vi "CSM - Running Log(Auto Filter Loop State) - DebugTool.vi"() -> ()   [LabVIEW 2017]
uses:
  _Support/Typedef/_CSM_GlobalLog_MSG.ctl
  _Support/Typedef/_CSM_Response Source Message.ctl
  _Support/Typedef/_CSM_GlobalLog_MSG_TYPE.ctl
  _Support/GlobalEvent/Gevt-ThreadQueueName.vi
  _Support/FGV-BroadcastRegistry/global-CSMQ FGV Change Flag.vi
  _Support/CSMQ/_CSMOFGV.vi
  Communicable State Machine.lvlib
  _Support/csm-tool-support.lvlib
  addons/Logger/CSM File Logger.lvlib
panel:
  in  "Record.Stop":bool
  in  "Record.Start":bool
  in  "BackTop":bool
  in  "Toolbar.History Length(char)":i32=100000 caption="History(char)" min=1000 max=100000000 step=1
  in  "Clear":bool
  in  "CSM":string(combo)
  in  "Search Button":bool
  in  "Toolbar.Open BD":bool
  in  "Toolbar.Open FP":bool
  out "State History":string
  in  "Tab":enum32{"Error History", "Broadcast Registry"}(tab)
  out "Error History":string
  out "Broadcast Registry":string[][](table)
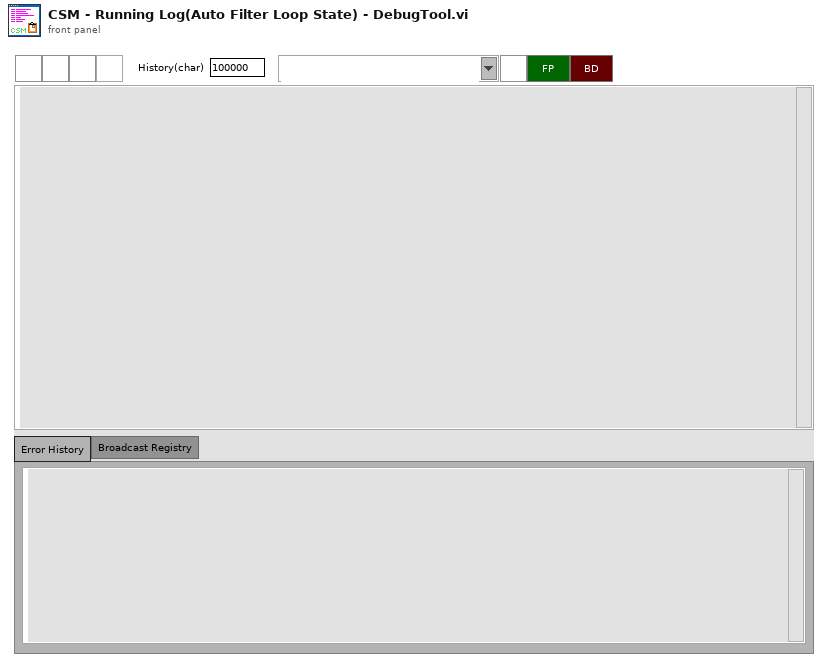
[diagram p1: front panel]
types:
  T1 = typedef "Communicable State Machine.lvlib/_CSM_GlobalLog_MSG.ctl" = cluster{"Name(\"\" to use uuid)":string, "Current State":string, "Arguments":string, "Source Message":T2, "Source Module":string, "Complete(T)/Start(F)":bool, "LogType":T3}
  T2 = typedef "Communicable State Machine.lvlib/_CSM_Response Source Message.ctl" = cluster{"‘State":string, "’Arguments":string, "’Error":errorcluster}
  T3 = typedef "Communicable State Machine.lvlib/_CSM_GlobalLog_MSG_TYPE.ctl" = enum16{"User Log", "State Change", "Status", "Interrupt", "Register", "Unregister", "Error Log", "Module Created", "Module Destroyed"}
  T4 = enum32{"Invalid", "Standard", "Closed", "Hidden", "Minimized", "Maximized"}
  T5 = enum32{"invalid app kind", "Development System", "Run Time System", "Student Edition", "Embedded LabVIEW", "Evaluation", "Custom"}
  T6 = cluster{"Shift":bool, "Ctrl":bool, "Alt":bool, "Cmd":bool, "Opt":bool}
  T7 = cluster{"Core":cluster{"Current VI Reference":refnum<vi>, "Close Panel on Exit?":bool}, "Toolbar.Advance":refnum<vi>[], "LoggerWatchDogQueue":refnum<queue>, "LogFile":path}
  T8 = cluster{"Current VI Reference":refnum<vi>, "Close Panel on Exit?":bool}
  T9 = typedef "Communicable State Machine.lvlib/CSM - Broadcast Message Type.ctl" = enum16{"Status", "Interrupt(High)"}
  T10 = cluster{"Status":string, "Source CSM":string, "Target CSM":string, "Target API":string, "Priority":T9}[]
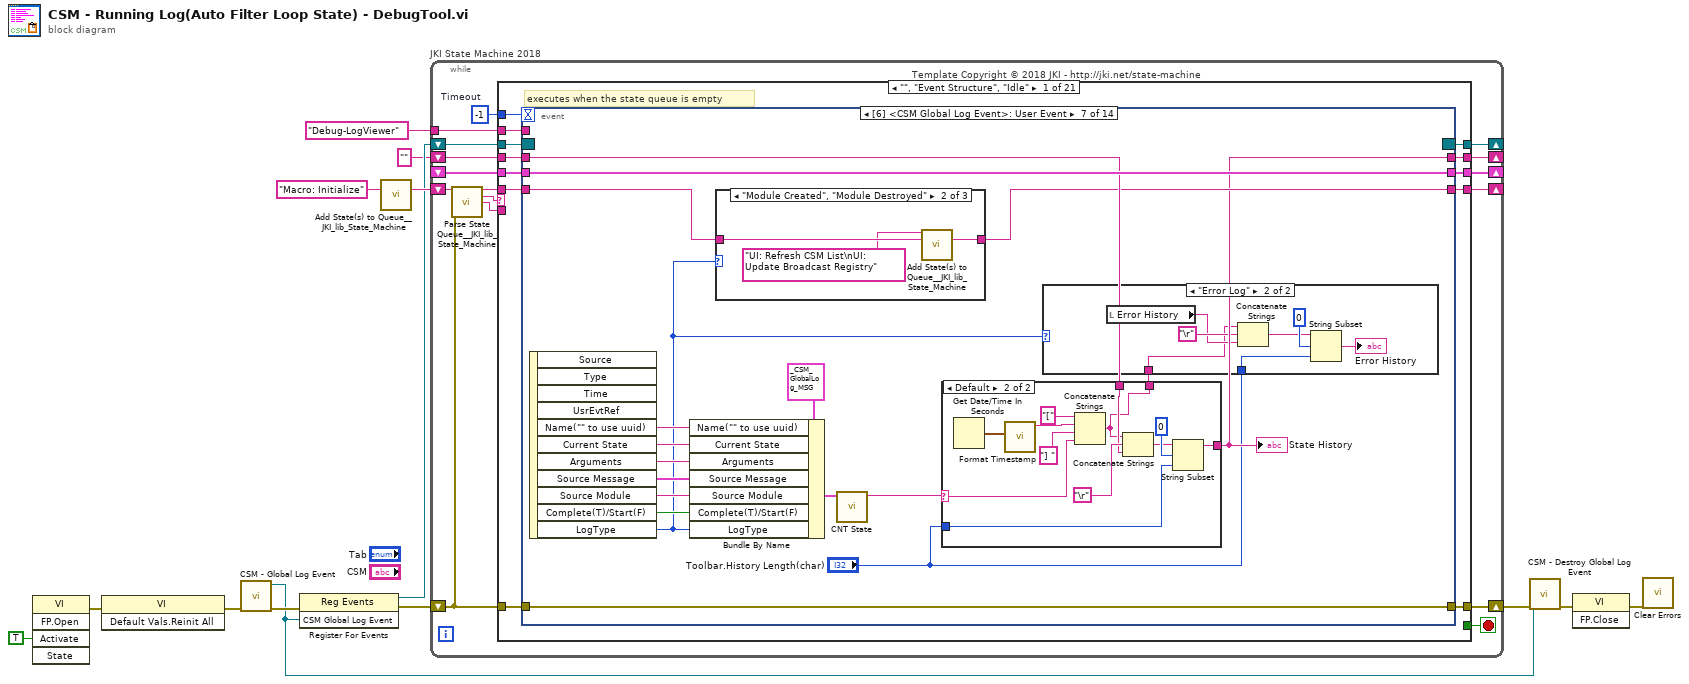
[diagram p0: block diagram]
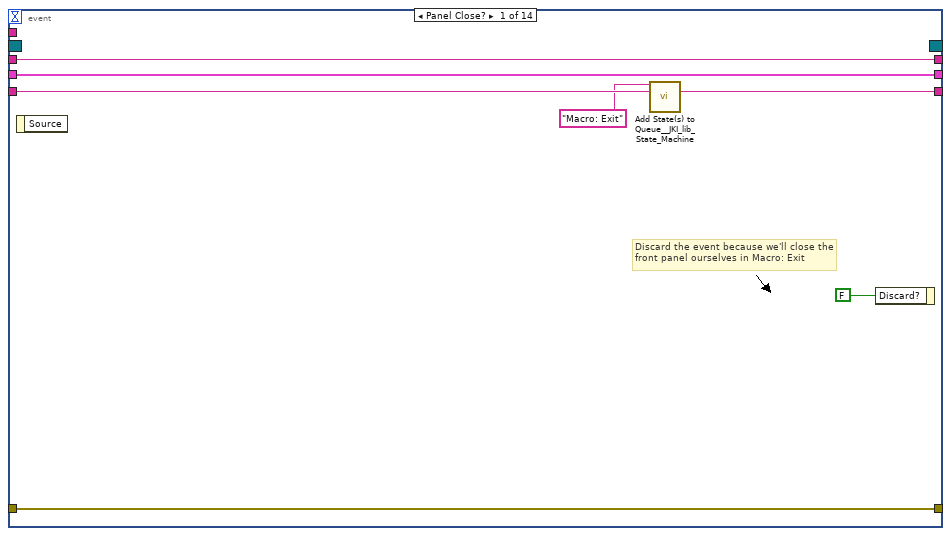
[diagram p2: hidden frame]
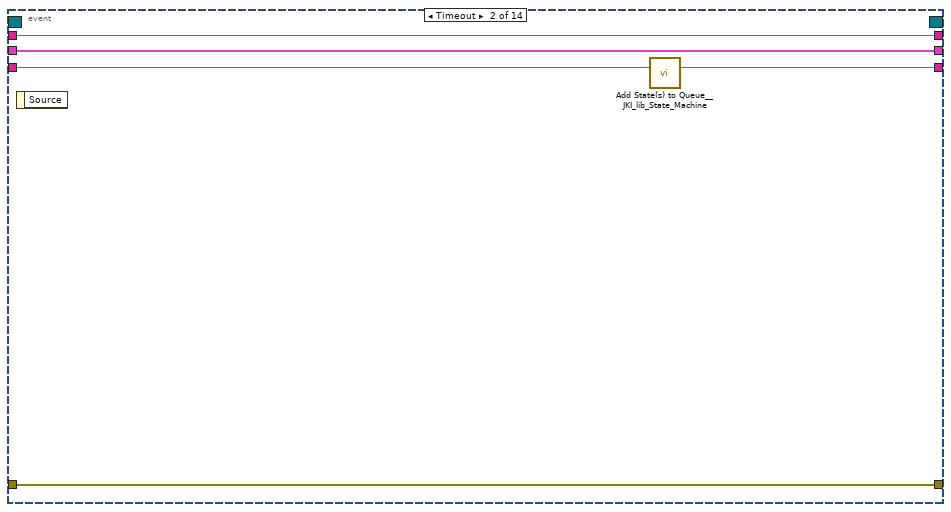
[diagram p3: hidden frame]
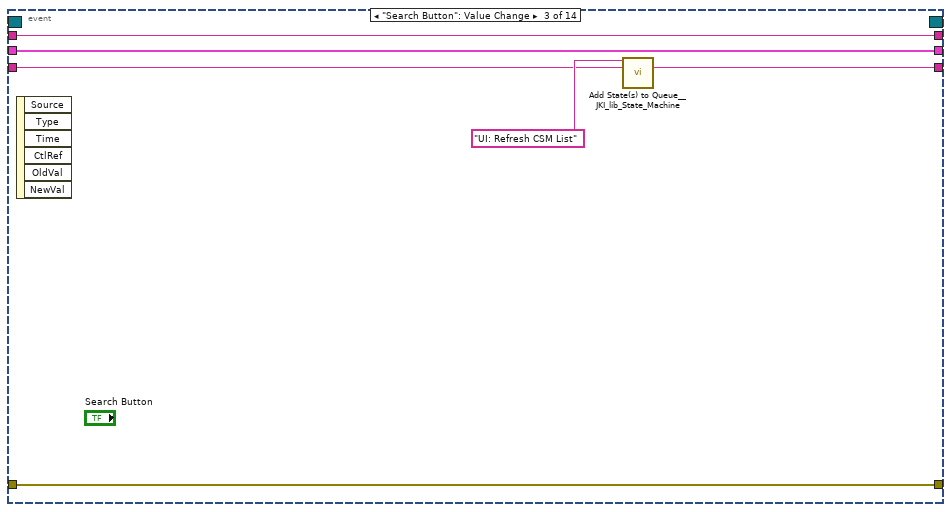
[diagram p4: hidden frame]
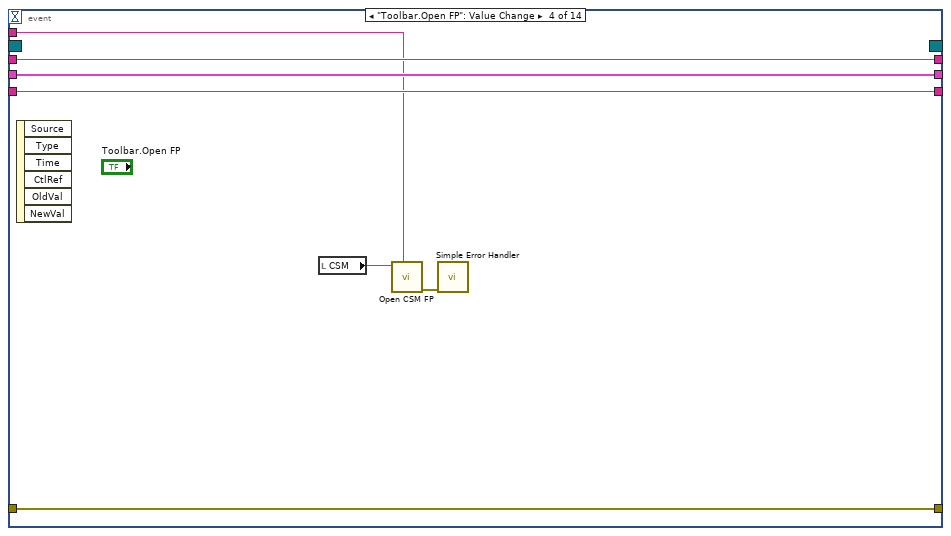
[diagram p5: hidden frame]
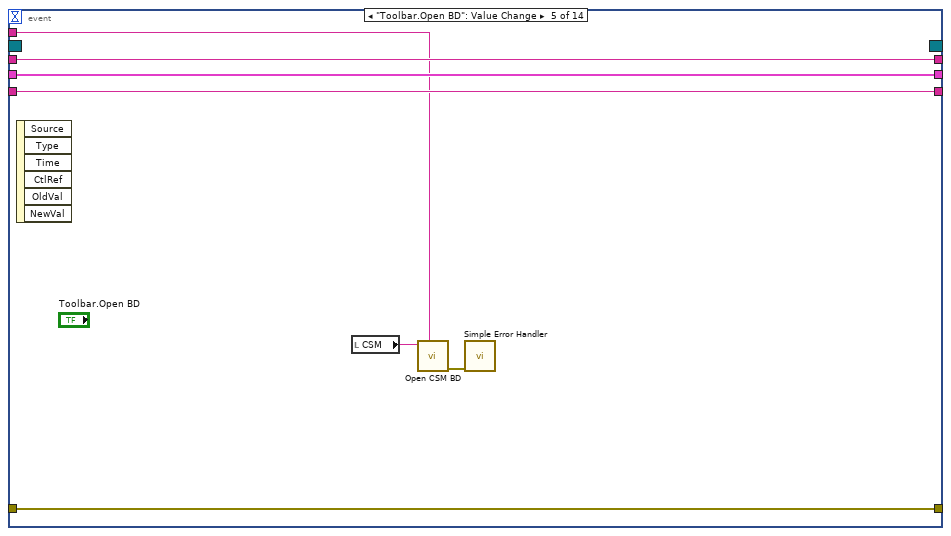
[diagram p6: hidden frame]
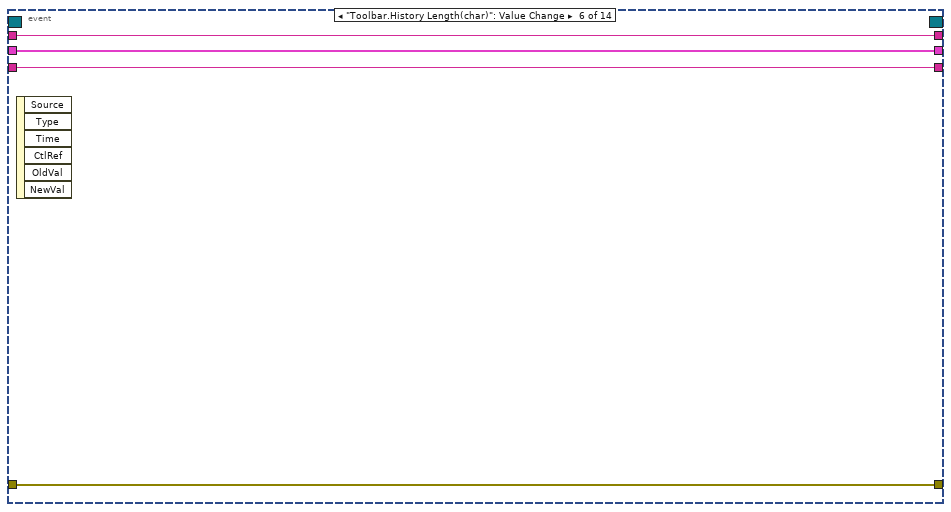
[diagram p7: hidden frame]
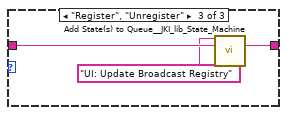
[diagram p10: hidden frame]
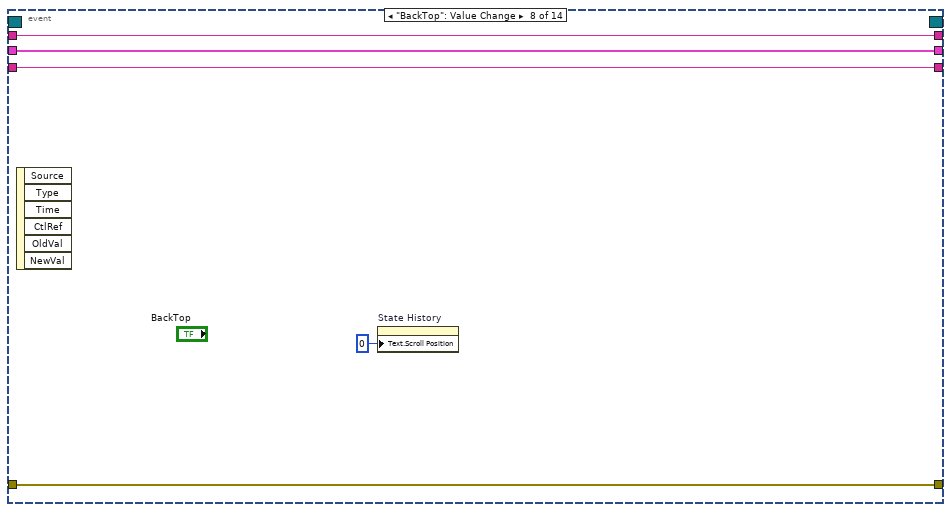
[diagram p12: hidden frame]
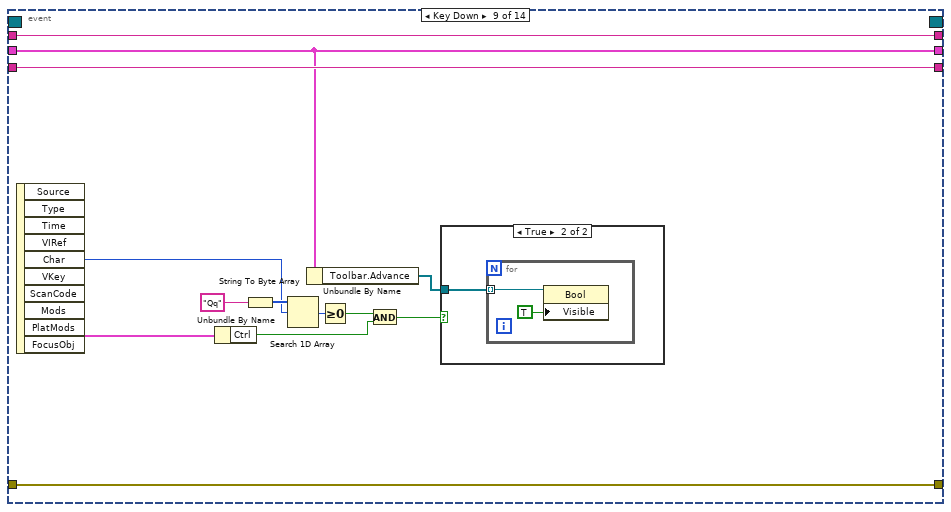
[diagram p13: hidden frame]
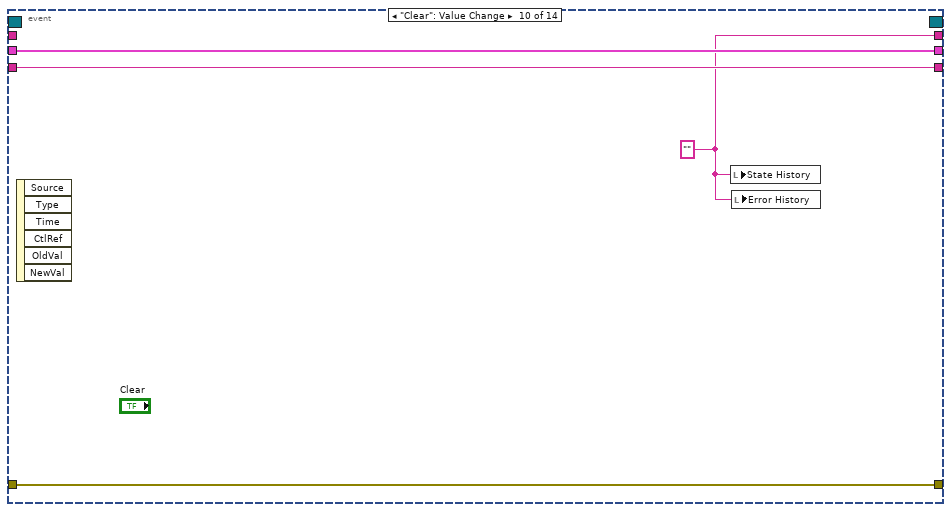
[diagram p15: hidden frame]
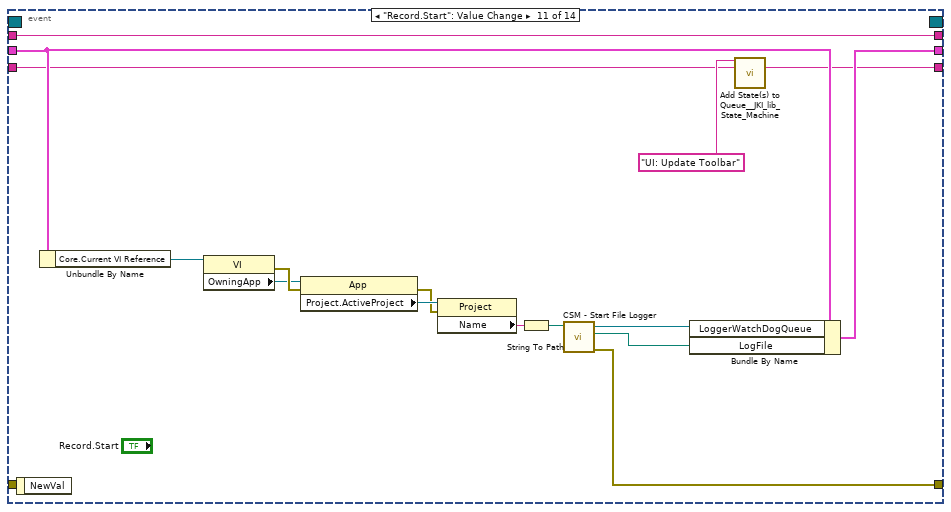
[diagram p16: hidden frame]
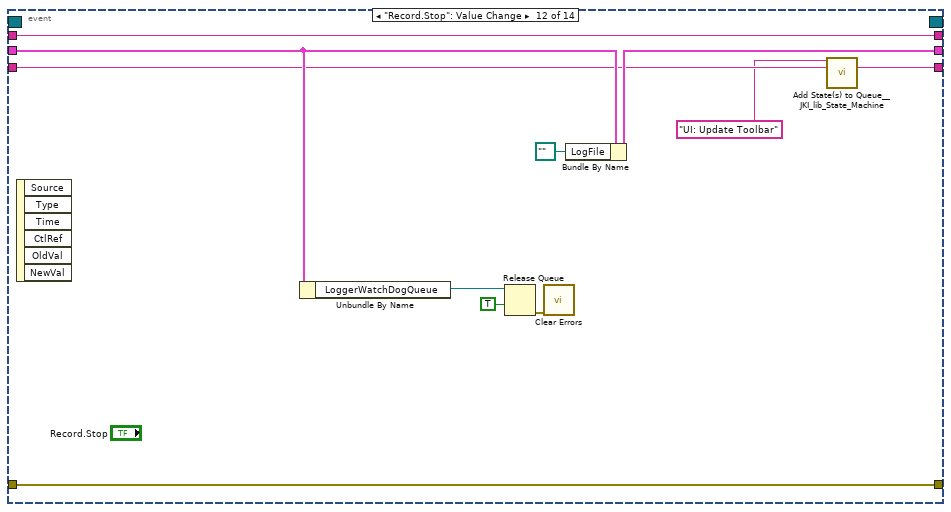
[diagram p17: hidden frame]
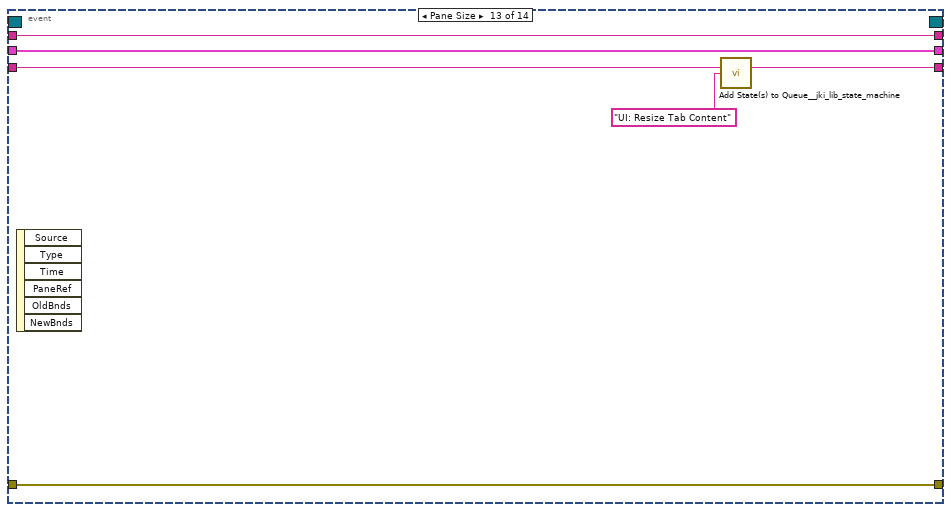
[diagram p18: hidden frame]
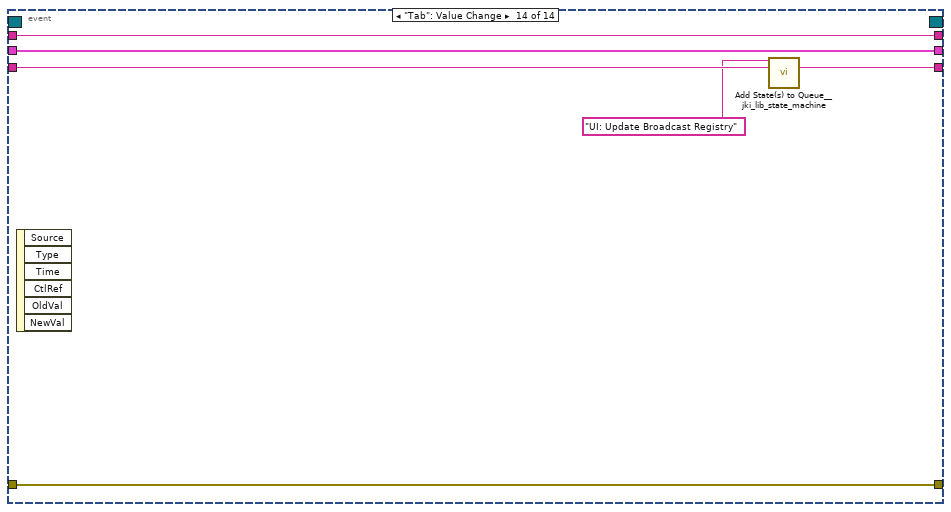
[diagram p19: hidden frame]
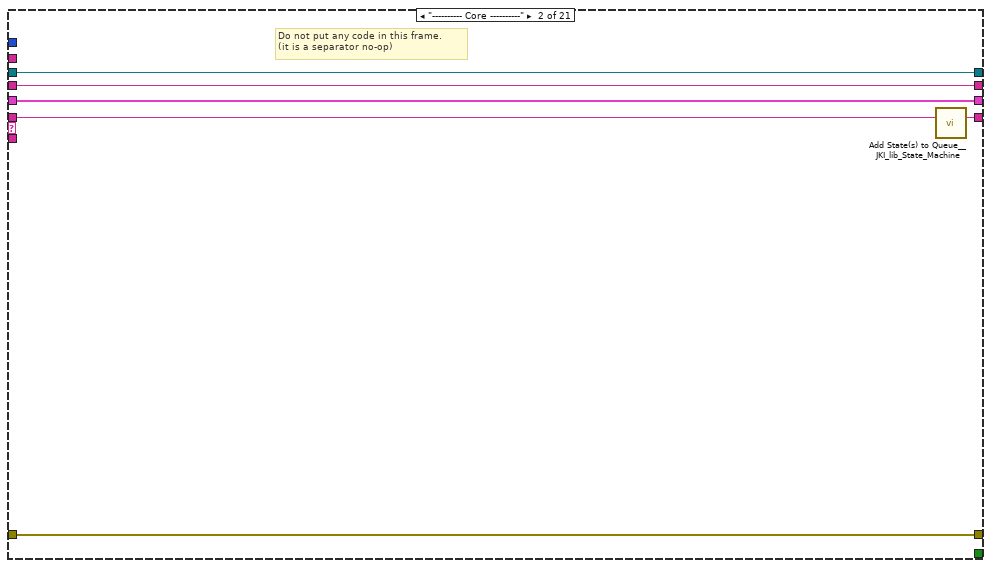
[diagram p20: hidden frame]
diagram:
  n1 = invoke class="VI" method="FP.Open"("Activate"=TRUE ("Activate?")) -> (error out=w13:errorcluster)  [unwired: 4 in, 4 out]
  n2 = invoke class="VI" method="Default Vals.Reinit All"(error in=w13) -> (error out=w7:errorcluster)  [unwired: 2 in, 2 out]
  n3 = call "CSM - Global Log Event.vi"("Error in"=w7) -> ("Error out"=w11:errorcluster, "CSM Global Log Event"=w10:refnum<user-event>)  [unwired: 9 in]
  n4 = register-events(error in=w11, w10) -> (reference out=w5:refnum<event-registration>, error out=w6:errorcluster)  [unwired: 1 in]
  n5 = call <vilib>:"Add State(s) to Queue__JKI_lib_State_Machine.vi"("State(s) in (\"\")"="Macro: Initialize") -> ("States Out"=w9:string)  [unwired: 14 in]
  n6 = while "JKI State Machine 2018" {
    shift-right: [w23] -> _
    shift-left: _ -> [w22]
    shift-right: [w26] -> w4
    shift-left: w6 -> [w20]
    shift-right: [w25] -> _
    shift-left: w9 -> [w27]
    shift-right: [w18] -> _
    shift-left: w5 -> [w19]
    tunnel: "Debug-LogViewer" ("Current Module(\"\" to generate a ID)") -> [w17]
    shift-right: [w15] -> _
    shift-left: "" ("String Cache") -> [w16]
    stop <- w24 stop-if-true
    w21 = -1  # Timeout
    # "Template Copyright © 2018 JKI - http://jki.net/state-machine"
    n7 = call <vilib>:"Parse State Queue__JKI_lib_State_Machine.vi"("State Queue"=w27, "Error In (no error)"=w20) -> ("Remaining States"=w29:string, "Current State"=w30:string, "Arguments"=w28:string)  [unwired: 11 in]
    n8 = case shown="\"\", \"Event Structure\", \"Idle\"" w30 {
      selector: w30 -> [_ _ w196 _ _ _ _ _ _ _ _ _ _ _ _ _ _ _ _ _ _]
      tunnel: w29 -> [w42 w193 w200 w221 w229 w236 w242 w252 w261 w269 w275 w282 w293 w306 w382 w389 w417 w440 w447 w454 w466]
      tunnel: w28 -> [_ _ _ _ _ _ _ _ _ _ _ _ w288 w300 _ _ _ _ _ _ _]
      tunnel: w22 -> [w40 w190 w198 w214 w226 w234 w239 _ w260 w264 w272 w277 w291 w302 w381 w388 w412 w439 w444 w451 w463]
      tunnel: [w39 w191 w202 w218 errorcluster {"status"=FALSE, "code"=0, "source"=""} ("error out") w233 w240 w249 w253 w265 w273 w280 w289 w303 w383 w390 w418 w441 w445 w452 w464] -> w26
      tunnel: w20 -> [w38 w191 w201 w218 w225 w233 w240 w249 w253 w266 w273 w280 w290 w304 w383 w390 w418 w441 w445 w452 w464]
      tunnel: [w41 w192 w199 w220 w228 w235 w241 w251 w261 w268 w274 w281 w292 w305 w382 w389 w417 w440 w446 w453 w465] -> w25
      tunnel: [_ _ _ _ _ TRUE _ _ _ _ _ _ _ _ _ _ _ _ _ _ _] -> w24
      tunnel: [w37 w190 w198 w219 w226 w234 w239 w250 w257 w264 w272 w277 w291 w302 w381 w388 w412 w439 w444 w451 w463] -> w23
      tunnel: w21 -> [w36 _ _ _ _ _ _ _ _ _ _ _ _ _ _ _ _ _ _ _ _]
      tunnel: w19 -> [w35 w189 w195 w208 w223 w231 w238 w247 w259 w263 w271 w279 w287 w299 w380 w387 w416 w438 w443 w449 w456]
      tunnel: [w34 w189 w195 w208 w223 w231 w238 w247 w259 w263 w271 w279 w287 w299 w380 w387 w416 w438 w443 w449 w456] -> w18
      tunnel: w17 -> [w33 _ _ _ _ _ _ _ _ _ _ _ _ _ _ _ _ _ _ _ _]
      tunnel: w16 -> [w32 w188 w194 w207 w222 w230 w237 w246 w258 w262 w270 w278 w286 w298 w379 w386 w415 w437 w442 w448 w455]
      tunnel: [w31 w188 w194 w207 w222 w230 w237 w246 w258 w262 w270 w278 w286 w298 w379 w386 w415 w437 w442 w448 w455] -> w15
      frame "", "Event Structure", "Idle" {
        # "executes when the state queue is empty"
        n9 = event shown="[6] <CSM Global Log Event>: User Event" {
          selector: w35 -> [_ _ _ _ _ _ _ _ _ _ _ _ _ _]
          dyn-events: [_ _ _ _ _ _ _ _ _ _ _ _ _ _] -> w34
          timeout: w36 -> [_ _ _ _ _ _ _ _ _ _ _ _ _ _]
          tunnel: w42 -> [w49 w54 w56 w66 w74 w78 w86 w128 w141 w148 w150 w167 w177 w183]
          tunnel: [w48 w53 w55 w66 w74 w78 w85 w128 w141 w148 w149 w166 w178 w184] -> w41
          tunnel: w40 -> [w46 w51 w60 w67 w72 w76 w95 w126 w131 w146 w159 w173 w180 w186]
          tunnel: [w47 w52 w59 w65 w73 w77 w96 w127 w140 w147 w161 w175 w181 w187] -> w39
          tunnel: w38 -> [w47 w52 w59 w65 w73 w77 w96 w127 w140 w147 _ w175 w181 w187]
          tunnel: [w46 w51 w60 w67 w72 w76 w95 w126 w131 w146 w162 w169 w180 w186] -> w37
          tunnel: w33 -> [_ _ _ w62 w69 _ _ _ _ _ _ _ _ _]
          tunnel: w32 -> [w43 w50 w58 w64 w71 w75 w87 w125 w139 _ w164 w174 w179 w185]
          tunnel: [w43 w50 w58 w64 w71 w75 w83 w125 w139 w145 w164 w174 w179 w185] -> w31
          event Panel Close? {
            # "Discard the event because we'll close the front panel ourselves in Macro: Exit"
            n10 = event-data() -> ()  [unwired: 1 in, 1 out]
            n11 = call <vilib>:"Add State(s) to Queue__JKI_lib_State_Machine.vi"("State(s) in Front (\"\")"="Macro: Exit", "State(s) in (\"\")"=w49) -> ("States Out"=w48:string)  [unwired: 13 in]
            n12 = event-data("Discard?"=FALSE) -> ()  [unwired: 1 in, 1 out]
          }
          event Timeout {
            n13 = event-data() -> ()  [unwired: 1 in, 1 out]
            n14 = call <vilib>:"Add State(s) to Queue__JKI_lib_State_Machine.vi"("State(s) in (\"\")"=w54) -> ("States Out"=w53:string)  [unwired: 14 in]
          }
          event "Search Button": Value Change {
            n15 = event-data() -> ()  [unwired: 1 in, 6 out]
            n16 = call <vilib>:"Add State(s) to Queue__JKI_lib_State_Machine.vi"("State(s) in Front (\"\")"="UI: Refresh CSM List" ("State(s) in Front (\"\")"), "State(s) in (\"\")"=w56) -> ("States Out"=w55:string)  [unwired: 13 in]
          }
          event "Toolbar.Open FP": Value Change {
            n17 = event-data() -> ()  [unwired: 1 in, 6 out]
            n18 = local read "CSM"() -> (w61:string)
            n19 = call "Open CSM FP.vi"("Current Module(\"\" to generate a ID)"=w62, "CSM"=w61) -> ("error out"=w63:errorcluster)  [unwired: 9 in]
            n20 = call <vilib>:"Simple Error Handler.vi"("error in (no error)"=w63) -> ()  [unwired: 4 in, 5 out]
          }
          event "Toolbar.Open BD": Value Change {
            n21 = event-data() -> ()  [unwired: 1 in, 6 out]
            n22 = local read "CSM"() -> (w68:string)
            n23 = call "Open CSM BD.vi"("Current Module(\"\" to generate a ID)"=w69, "CSM"=w68) -> ("error out"=w70:errorcluster)  [unwired: 9 in]
            n24 = call <vilib>:"Simple Error Handler.vi"("error in (no error)"=w70) -> ()  [unwired: 4 in, 5 out]
          }
          event "Toolbar.History Length(char)": Value Change {
            n25 = event-data() -> ()  [unwired: 1 in, 6 out]
          }
          event User Event {
            n26 = event-data() -> ("Name(\"\" to use uuid)"=w93:string, "Current State"=w92:string, "Arguments"=w91:string, "Source Message"=w90:T2, "Source Module"=w89:string, "Complete(T)/Start(F)"=w88:bool, "LogType"=w84:T3)  [unwired: 1 in, 4 out]
            n27 = Bundle By Name(cluster=T1 {"Name(\"\" to use uuid)"="", "Current State"="", "Arguments"="", "Source Message"={"‘State"="", "’Arguments"="", "’Error"={"status"=FALSE, "code"=0, "source"=""}}, "Source Module"="", "Complete(T)/Start(F)"=FALSE, "LogType"=enum."State Change"} ("Cross CSM Data"), "Name(\"\" to use uuid)"=w93, "Current State"=w92, "Arguments"=w91, "Source Message"=w90, "Source Module"=w89, "Complete(T)/Start(F)"=w88, "LogType"=w84) -> (w80:T1)
            n28 = case shown="\"Module Created\", \"Module Destroyed\"" w84 {
              tunnel: w86 -> [w104 w107 w110]
              tunnel: [w104 w106 w109] -> w85
              frame "User Log", Default {
              }
              frame "Module Created", "Module Destroyed" {
                n29 = call <vilib>:"Add State(s) to Queue__JKI_lib_State_Machine.vi"("State(s) in Front (\"\")"="UI: Refresh CSM List\nUI: Update Broadcast Registry" ("State(s) in Front (\"\")"), "State(s) in (\"\")"=w107) -> ("States Out"=w106:string)  [unwired: 13 in]
              }
              frame "Register", "Unregister" {
                n30 = call <vilib>:"Add State(s) to Queue__JKI_lib_State_Machine.vi"("State(s) in Front (\"\")"="UI: Update Broadcast Registry" ("State(s) in Front (\"\")"), "State(s) in (\"\")"=w110) -> ("States Out"=w109:string)  [unwired: 13 in]
              }
            }
            n31 = call "CNT State.vi"("Cross CSM Data"=w80) -> ("Log String"=w79:string)  [unwired: 9 in, 1 out]
            n32 = case shown="Default" w79 {
              selector: w79 -> [_ w123]
              tunnel: [w111 w121] -> w83
              tunnel: "Toolbar.History Length(char)" -> [_ w120]
              tunnel: w87 -> [w111 w115]
              tunnel: [_ w114] -> w81
              frame "" {
              }
              frame Default {
                n33 = Get Date/Time In Seconds() -> (seconds since 1Jan1904=w112:timestamp)
                n34 = call "Format Timestamp.vi"("timestamp"=w112) -> ("String"=w113:string)  [unwired: 10 in]
                n35 = Concatenate Strings("[" ("string"), w113, "] " ("string"), w123) -> (w114:string)
                n36 = Concatenate Strings(w114, "\r", w115) -> (w117:string)
                n37 = String Subset(string=w117, offset (0)=0, length (rest)=w120) -> (substring=w121:string)
              }
            }
            "State History" <- w83
            n38 = case shown="\"Error Log\"" w84 {
              tunnel: "Toolbar.History Length(char)" -> [_ w98]
              tunnel: w81 -> [_ w97]
              frame "User Log", Default {
              }
              frame "Error Log" {
                n39 = local read "Error History"() -> (w102:string)
                n40 = Concatenate Strings(w97, "\r", w102) -> (w100:string)
                n41 = String Subset(string=w100, offset (0)=0, length (rest)=w98) -> (substring=→"Error History":string)
              }
            }
          }
          event "BackTop": Value Change {
            n42 = event-data() -> ()  [unwired: 1 in, 6 out]
            n43 = property on="State History" class="Str"("Text.Scroll Position"=u32 0) -> ()  [unwired: 2 in, 2 out]
          }
          event Key Down {
            n44 = event-data() -> ("Char"=w129:i16, "PlatMods"=w134:T6)  [unwired: 1 in, 8 out]
            n45 = Unbundle By Name(w134) -> ("Ctrl"=w133:bool)
            n46 = String To Byte Array(string="Qq") -> (unsigned byte array=w136:u8[])
            n47 = Search 1D Array(1D array=w136, element=w129) -> (index of element=w137:i32)  [unwired: 1 in]
            n48 = Unbundle By Name(w131) -> ("Toolbar.Advance"=w130:refnum<vi>[])
            n49 = Greater Or Equal To 0?(x=w137) -> (x >= 0?=w138:bool)
            n50 = And(x=w138, y=w133) -> (x .and. y?=w132:bool)
            n51 = case shown="True" w132 {
              tunnel: w130 -> [_ w142]
              frame False {
              }
              frame True {
                n52 = for {
                  tunnel: w142 -> [w144] mode=indexing
                  n53 = property class="Bool"(reference=w144, "Visible"=TRUE) -> ()  [unwired: 1 in, 2 out]
                }
              }
            }
          }
          event "Clear": Value Change {
            w145 = "" ("String Cache")
            n54 = event-data() -> ()  [unwired: 1 in, 6 out]
            n55 = local write "State History"(w145) -> ()
            n56 = local write "Error History"(w145) -> ()
          }
          event "Record.Start": Value Change {
            n57 = event-data() -> ()  [unwired: 1 in, 1 out]
            n58 = Unbundle By Name(w159) -> ("Core.Current VI Reference"=w158:refnum<vi>)
            n59 = property class="VI"(reference=w158) -> (error out=w157:errorcluster, "OwningApp"=w156:refnum<vi>)  [unwired: 1 in, 1 out]
            n60 = property class="App"(reference=w156, error in=w157) -> (error out=w154:errorcluster, "Project.ActiveProject"=w155:refnum<vi>)  [unwired: 1 out]
            n61 = property class="Project"(reference=w155, error in=w154) -> ("Name"=w153:string)  [unwired: 2 out]
            n62 = String To Path(string=w153) -> (path=w152:path)
            n63 = call "CSM - Start File Logger.vi"("Log File Path"=w152) -> ("Error out"=w161:errorcluster, "LogFile"=w160:path, "WatchDogQueue"=w163:refnum<queue>)  [unwired: 8 in]
            n64 = Bundle By Name(cluster=w159, "LoggerWatchDogQueue"=w163, "LogFile"=w160) -> (w162:T7)
            n65 = call <vilib>:"Add State(s) to Queue__JKI_lib_State_Machine.vi"("State(s) in Front (\"\")"="UI: Update Toolbar" ("State(s) in Front (\"\")"), "State(s) in (\"\")"=w150) -> ("States Out"=w149:string)  [unwired: 13 in]
          }
          event "Record.Stop": Value Change {
            n66 = event-data() -> ()  [unwired: 1 in, 6 out]
            n67 = Unbundle By Name(w173) -> ("LoggerWatchDogQueue"=w172:refnum<queue>)
            n68 = Release Queue(queue=w172, force destroy? (F)=TRUE) -> (error out=w170:errorcluster)  [unwired: 1 in, 2 out]
            n69 = call <vilib>:"Clear Errors.vi"("error in (no error)"=w170) -> ()  [unwired: 5 in, 2 out]
            n70 = Bundle By Name(cluster=w173, "LogFile"=path "") -> (w169:T7)
            n71 = call <vilib>:"Add State(s) to Queue__JKI_lib_State_Machine.vi"("State(s) in Front (\"\")"="UI: Update Toolbar" ("State(s) in Front (\"\")"), "State(s) in (\"\")"=w167) -> ("States Out"=w166:string)  [unwired: 13 in]
          }
          event Pane Size {
            n72 = event-data() -> ()  [unwired: 1 in, 6 out]
            n73 = call <vilib>:"Add State(s) to Queue__jki_lib_state_machine.vi"("State(s) in (\"\")"=w177, "State(s) at Back (\"\")"="UI: Resize Tab Content" ("State(s) in Front (\"\")")) -> ("States Out"=w178:string)  [unwired: 13 in]
          }
          event "Tab": Value Change {
            n74 = event-data() -> ()  [unwired: 1 in, 6 out]
            n75 = call <vilib>:"Add State(s) to Queue__jki_lib_state_machine.vi"("State(s) in Front (\"\")"="UI: Update Broadcast Registry" ("State(s) in Front (\"\")"), "State(s) in (\"\")"=w183) -> ("States Out"=w184:string)  [unwired: 13 in]
          }
        }
      }
      frame "---------- Core ----------" {
        # "Do not put any code in this frame.\n(it is a separator no-op)"
        n76 = call <vilib>:"Add State(s) to Queue__JKI_lib_State_Machine.vi"("State(s) in (\"\")"=w193) -> ("States Out"=w192:string)  [unwired: 14 in]
      }
      frame Default {
        w205 = 42 items=["No error", "Argument error", "Memory is full", "Out of zone", "End of file", "File already open", "Generic file I/O error", "File not found", "File permission error", "Disk is full", "Duplicate path", "Too many files open", "System feature not enabled", "Resource file not found", "Cannot add resource", "Resource not found", "Image not found", "Image memory error", "Pen does not exist", "Config type invalid", "Config token not found", "Config parse error", "Config memory error", "Bad external code format", "Bad external code offset", "External code not present", "Null window", "Destroy window error", "Null menu", "Print aborted", "Bad print record", "Print driver error", "Windows error during printing", "Memory error during printing", "Print dialog error", "Generic print error", "Invalid device refnum", "Device not found", "Device parameter error", "Device unit error", "Cannot open device", "Device call aborted", "Generic error", "Cancelled by user", "Object ID too low", "Object ID too high", "Object not in heap", "Unknown heap", "Unknown object (invalid DefProc)", "Unknown object (DefProc not in table)", "Message out of range", "Invalid (null) method", "Unknown message", "Manager call not supported", "Bad address", "Network operation in progress", "Network operation timed out", "Connection is busy", "Network attribute not supported", "Network error", "Address in use", "System out of memory", "Connection aborted", "Connection refused", "Not connected", "Already connected", "Connection closed", "Initialization error (interapplication manager)", "Bad occurrence", "Wait on unbound occurrence handler", "Occurrence queue overflow", "Datalog type conflict", "Unused", "Unrecognized type (interapplication manager)", "Memory corrupt", "Failed to make temporary DLL", "Old CIN version", "Drag socket not found", "Failed to load drop-object", "Failed to register OLE object", "Failed to release OLE object", "Format specifier type mismatch", "Unknown format specifier", "Too few format specifiers", "Too many format specifiers", "Scan failed", "Newer CIN version", "Error converting to variant", "Runtime menu error", "Password tampered", "Variant attribute not found", "Incompatible variant data type", "Event data is not available", "Event Store is not present", "Occurrence is not found", "Event Queue is not created", "Event info is not available", "Refnum passed is NULL", "Error retrieving Class GUID", "Error retrieving CoClass GUID", "Error retrieving TypeLib GUID.", "Bad built application magic bytes.", "Specific driver is different from the specific driver associated with the Logical Name.", "There is no session opened to the class driver.", "Max Error", "MAX - Error with config objects", "MAX - Error loading configuration", "MAX - Group not supported"]
        # "Current State"
        # "Do not delete, rename, or modify this frame.\n(this is used to capture unhandled states and typos)"
        # "Handle mistyped state name (developer tool)"
        n77 = Format Into String(format string="Software Exception: Unhandled State \"%s\"." ("message"), error in=w201, w196) -> (resulting string=w204:string, error out=w203:errorcluster)  [unwired: 1 in]
        n78 = call <vilib>:"Error Cluster From Error Code.vi"("show call chain? (False)"=TRUE, "error in (no error)"=w203, "error message (\"\")"=w204, "error code (0)"=w205) -> ("error out"=w202:errorcluster)  [unwired: 5 in]
        n79 = call <vilib>:"Add State(s) to Queue__JKI_lib_State_Machine.vi"("State(s) in (\"\")"=w200) -> ("States Out"=w199:string)  [unwired: 14 in]
      }
      frame "Initialize Core Data" {
        # "Do not delete, rename, or modify this frame.\n(this is used to determine panel behavior on exit)"
        # "originally closed?"
        # "exe?"
        # "If panel starts closed or is an EXE, then close it when we exit"
        n80 = property class="VI"() -> ("FP.State"=w211:T4)  [unwired: 2 in, 2 out]
        n81 = property class="App"() -> ("App.Kind"=w217:T5)  [unwired: 2 in, 2 out]
        n82 = control-ref of="Current VI Reference"() -> (w212:refnum<vi>)
        n83 = Equal?(x=w211, y=T4."Closed" ("Front Panel Window:State")) -> (x = y?=w209:bool)
        n84 = Equal?(x=w217, y=T5."Run Time System" ("Application:Kind")) -> (x = y?=w215:bool)
        n85 = Or(x=w209, y=w215) -> (x .or. y?=w213:bool)
        n86 = Bundle By Name(cluster=w214, "Core.Current VI Reference"=w212, "Core.Close Panel on Exit?"=w213) -> (w219:T7)
        n87 = call <vilib>:"Add State(s) to Queue__JKI_lib_State_Machine.vi"("State(s) in (\"\")"=w221) -> ("States Out"=w220:string)  [unwired: 14 in]
      }
      frame "Error Handler" {
        # "Unhandled Error -- Display it"
        # "Handle any errors here.\nYou can also output any states to clean-up after errors occur"
        # "Clear error"
        n88 = call <vilib>:"General Error Handler.vi"("error in (no error)"=w225) -> ()  [unwired: 10 in, 5 out]
        n89 = call <vilib>:"Add State(s) to Queue__JKI_lib_State_Machine.vi"("State(s) in Front (\"\")"="/* Post Error States", "State(s) in (\"\")"=w229) -> ("States Out"=w228:string)  [unwired: 13 in]
      }
      frame "Exit" {
        # "Do not put any code in this frame.\n(No errors that occur here will be handled.)"
        n90 = call <vilib>:"Add State(s) to Queue__JKI_lib_State_Machine.vi"("State(s) in (\"\")"=w236) -> ("States Out"=w235:string)  [unwired: 14 in]
      }
      frame "---------- Data ----------" {
        # "Do not put any code in this frame.\n(It is a separator no-op. You can make a copy of this frame to create a new Data frame)"
        n91 = call <vilib>:"Add State(s) to Queue__JKI_lib_State_Machine.vi"("State(s) in (\"\")"=w242) -> ("States Out"=w241:string)  [unwired: 14 in]
      }
      frame "Data: Initialize" {
        w243 = refnum<queue> refnum  # LoggerWatchDogQueue
        w244 = path ""  # LogFile
        w245 = refnum<vi>[] []  # Toolbar.Advance
        w248 = T8 {"Current VI Reference"=refnum, "Close Panel on Exit?"=FALSE}  # Core
        # "Data names and types of shift register data are defined by this bundle."
        # "Initialize the shift-register data, here.\n(data names are defined by what you wire into the bundle function)"
        n92 = Bundle("Core"=w248, "Toolbar.Advance"=w245, "LoggerWatchDogQueue"=w243, "LogFile"=w244) -> (w250:T7)  [unwired: 1 in]
        n93 = call <vilib>:"Add State(s) to Queue__JKI_lib_State_Machine.vi"("State(s) in (\"\")"=w252) -> ("States Out"=w251:string)  [unwired: 14 in]
      }
      frame "Data: Initialize References" {
        n94 = control-ref of="Toolbar.Open BD"() -> (w255:refnum<vi>)
        n95 = control-ref of="Toolbar.Open FP"() -> (w256:refnum<vi>)
        n96 = Build Array(w255, w256) -> (w254:refnum<vi>[])
        n97 = Bundle By Name(cluster=w260, "Toolbar.Advance"=w254) -> (w257:T7)
      }
      frame "Data: Cleanup" {
        # "Cleanup any data and references, here.\n(this is called automatically, by the Macro: Exit)"
        n98 = Unbundle By Name(w264) -> ("Core.Current VI Reference"=w267:refnum<vi>)
        n99 = Close Reference(reference=w267, error in (no error)=w266) -> (error out=w265:errorcluster)
        n100 = call <vilib>:"Add State(s) to Queue__JKI_lib_State_Machine.vi"("State(s) in (\"\")"=w269) -> ("States Out"=w268:string)  [unwired: 14 in]
      }
      frame "---------- UI ----------" {
        # "Do not put any code in this frame.\n(It is a separator no-op. You can make a copy of this frame to create a new UI frame)"
        n101 = call <vilib>:"Add State(s) to Queue__JKI_lib_State_Machine.vi"("State(s) in (\"\")"=w275) -> ("States Out"=w274:string)  [unwired: 14 in]
      }
      frame "UI: Initialize" {
        # "Initialize the User Interface, here.\n(this is called automatically, by the Macro: Init)"
        n102 = Unbundle By Name(w277) -> ("Toolbar.Advance"=w276:refnum<vi>[])
        n103 = disable-structure shown="Disabled" {
          disable-tunnel: w276 -> [w283 _]
          frame Disabled {
            n104 = for {
              tunnel: w283 -> [w285] mode=indexing
              n105 = property class="Bool"(reference=w285, "Visible"=FALSE) -> ()  [unwired: 1 in, 2 out]
            }
          }
          frame Enabled {
          }
        }
        n106 = call <vilib>:"Add State(s) to Queue__JKI_lib_State_Machine.vi"("State(s) in (\"\")"=w282) -> ("States Out"=w281:string)  [unwired: 14 in]
      }
      frame "UI: Cursor Set" {
        # "Argument"
        # "Set and Unset Cursor Busy.\n(Usage: \"UI: Cursor Set >> Busy|Idle\")"
        n107 = case shown="\"Idle\", Default" w288 {
          tunnel: w290 -> [w295 w297]
          tunnel: [w294 w296] -> w289
          frame "Idle", Default {
            n108 = call <vilib>:"Unset Busy.vi"("error in (no error)"=w295) -> ("error out"=w294:errorcluster)  [unwired: 10 in]
          }
          frame "Busy" {
            n109 = call <vilib>:"Set Busy.vi"("error in (no error)"=w297) -> ("error out"=w296:errorcluster)  [unwired: 9 in, 1 out]
          }
        }
        n110 = call <vilib>:"Add State(s) to Queue__JKI_lib_State_Machine.vi"("State(s) in (\"\")"=w293) -> ("States Out"=w292:string)  [unwired: 14 in]
      }
      frame "UI: Front Panel State" {
        # "Argument"
        # "Set Front Panel Open or Closed\n(Usage: \"UI: Front Panel State >> Open|Close\")"
        n111 = Unbundle By Name(w302) -> ("Core.Current VI Reference"=w301:refnum<vi>)
        n112 = case shown="\"Minimize\", \"Minimized\"" w300 {
          tunnel: w304 -> [w312 w327 w338 w351 w364]
          tunnel: [w314 w328 w340 w353 w366] -> w303
          tunnel: w301 -> [w313 w325 w339 w352 w365]
          frame "Open", "Standard", Default {
            w307 = T4."Standard" ("State")
            n113 = property class="VI"(reference=w313, error in=w312) -> (reference out=w310:refnum<vi>, error out=w311:errorcluster, "FP.State"=w309:T4)
            n114 = Not Equal?(x=w309, y=w307) -> (x != y?=w308:bool)
            n115 = case shown="True" w308 {
              tunnel: [w318 w320] -> w314
              tunnel: w311 -> [w317 w320]
              tunnel: w310 -> [w316 _]
              tunnel: w307 -> [w315 _]
              frame True {
                n116 = invoke class="VI" method="FP.Open"(reference=w316, error in=w317, "Activate"=TRUE, "State"=w315) -> (error out=w318:errorcluster)  [unwired: 1 in, 4 out]
              }
              frame False {
              }
            }
          }
          frame "Close", "Closed" {
            n117 = property class="VI"(reference=w325, error in=w327) -> (reference out=w324:refnum<vi>, error out=w326:errorcluster, "FP.State"=w322:T4)
            n118 = Not Equal?(x=w322, y=T4."Closed" ("Front Panel Window:State")) -> (x != y?=w321:bool)
            n119 = case shown="True" w321 {
              tunnel: [w329 w332] -> w328
              tunnel: w326 -> [w329 w331]
              tunnel: w324 -> [_ w330]
              frame False {
              }
              frame True {
                n120 = invoke class="VI" method="FP.Close"(reference=w330, error in=w331) -> (error out=w332:errorcluster)  [unwired: 1 in, 2 out]
              }
            }
          }
          frame "Hidden", "Hide" {
            w333 = T4."Hidden" ("State")
            n121 = property class="VI"(reference=w339, error in=w338) -> (reference out=w336:refnum<vi>, error out=w337:errorcluster, "FP.State"=w335:T4)
            n122 = Not Equal?(x=w335, y=w333) -> (x != y?=w334:bool)
            n123 = case shown="True" w334 {
              tunnel: [w344 w345] -> w340
              tunnel: w337 -> [w343 w345]
              tunnel: w336 -> [w342 _]
              tunnel: w333 -> [w341 _]
              frame True {
                n124 = invoke class="VI" method="FP.Open"(reference=w342, error in=w343, "State"=w341) -> (error out=w344:errorcluster)  [unwired: 2 in, 4 out]
              }
              frame False {
              }
            }
          }
          frame "Minimize", "Minimized" {
            w346 = T4."Minimized" ("State")
            n125 = property class="VI"(reference=w352, error in=w351) -> (reference out=w349:refnum<vi>, error out=w350:errorcluster, "FP.State"=w348:T4)
            n126 = Not Equal?(x=w348, y=w346) -> (x != y?=w347:bool)
            n127 = case shown="True" w347 {
              tunnel: [w357 w358] -> w353
              tunnel: w350 -> [w356 w358]
              tunnel: w349 -> [w355 _]
              tunnel: w346 -> [w354 _]
              frame True {
                n128 = invoke class="VI" method="FP.Open"(reference=w355, error in=w356, "State"=w354) -> (error out=w357:errorcluster)  [unwired: 2 in, 4 out]
              }
              frame False {
              }
            }
          }
          frame "Maximize", "Maximized" {
            w359 = T4."Maximized" ("State")
            n129 = property class="VI"(reference=w365, error in=w364) -> (reference out=w362:refnum<vi>, error out=w363:errorcluster, "FP.State"=w361:T4)
            n130 = Not Equal?(x=w361, y=w359) -> (x != y?=w360:bool)
            n131 = case shown="True" w360 {
              tunnel: [w370 w371] -> w366
              tunnel: w363 -> [w369 w371]
              tunnel: w362 -> [w368 _]
              tunnel: w359 -> [w367 _]
              frame True {
                n132 = invoke class="VI" method="FP.Open"(reference=w368, error in=w369, "State"=w367) -> (error out=w370:errorcluster)  [unwired: 2 in, 4 out]
              }
              frame False {
              }
            }
          }
        }
        n133 = call <vilib>:"Add State(s) to Queue__JKI_lib_State_Machine.vi"("State(s) in (\"\")"=w306) -> ("States Out"=w305:string)  [unwired: 14 in]
      }
      frame "UI: Refresh CSM List" {
        n134 = property on="CSM" class="CmbBox"() -> ("Value"=w375:string)  [unwired: 2 in, 2 out]
        n135 = call "CSM - List Modules.vi"() -> ("Error out"=w372:errorcluster, "Module Names"=w377:string[])  [unwired: 10 in]
        n136 = Search 1D Array(1D array=w377, element=w375) -> (index of element=w373:i32)  [unwired: 1 in]
        n137 = Greater Or Equal To 0?(x=w373) -> (x >= 0?=w374:bool)
        n138 = Index Array(array=w377) -> (element=w376:string)  [unwired: 1 in]
        n139 = Select(t=w375, s=w374, f=w376) -> (s? t:f=w378:string)
        n140 = property on="CSM" class="CmbBox"("Strings[]"=w377, "Value"=w378) -> ()  [unwired: 2 in, 2 out]
        n141 = call <vilib>:"Simple Error Handler.vi"("error in (no error)"=w372) -> ()  [unwired: 4 in, 5 out]
      }
      frame "UI: Update Broadcast Registry" {
        n142 = call "CSM - List Mapping Relationships in Broadcast Registry.vi"() -> ("Array"=w384:T10)  [unwired: 10 in, 1 out]
        n143 = for {
          tunnel: w384 -> [w398] mode=indexing
          tunnel: [w391] -> w385 mode=indexing
          n144 = Unbundle(w398) -> ("Status"=w397:string, "Source CSM"=w396:string, "Target CSM"=w395:string, "Target API"=w394:string, "Priority"=w393:T9)
          n145 = Format Into String(w393) -> (resulting string=w392:string)  [unwired: 3 in, 1 out]
          n146 = Build Array(w397, w396, w395, w394, w392) -> (w391:string[])
        }
        "Broadcast Registry" <- w385
      }
      frame "UI: Update Toolbar" {
        w406 = i16 2 ("x")
        n147 = control-ref of="Record.Start"() -> (w414:refnum<vi>)
        n148 = control-ref of="Record.Stop"() -> (w413:refnum<vi>)
        n149 = Unbundle By Name(w412) -> ("Core.Current VI Reference"=w403:refnum<vi>, "LogFile"=w400:path, "LoggerWatchDogQueue"=w411:refnum<queue>)
        n150 = Not A Number/Path/Refnum?(number/path/refnum=w411) -> (NaN/Path/Refnum?=w404:bool)
        n151 = Not(x=w404) -> (.not. x?=w405:bool)
        n152 = Boolean To (0,1)(Boolean=w405) -> (0, 1=w410:i16)
        n153 = Boolean To (0,1)(Boolean=w404) -> (0, 1=w409:i16)
        n154 = Multiply(x=w406, y=w409) -> (x*y=w407:i16)
        n155 = Multiply(x=w406, y=w410) -> (x*y=w408:i16)
        n156 = Empty String/Path?(string/path=w400) -> (empty?=w399:bool)
        n157 = property class="Bool"(reference=w414, "DisabledEnum"=w408) -> ()  [unwired: 1 in, 2 out]
        n158 = property class="Bool"(reference=w413, "DisabledEnum"=w407) -> ()  [unwired: 1 in, 2 out]
        n159 = case shown="True" w399 {
          tunnel: "Running Log Viewer (CSM)" ("Front Panel Window:Title") -> [w423 w424]
          tunnel: [w422 w424] -> w401
          tunnel: w400 -> [w419 _]
          frame False {
            n160 = Path To String(path=w419) -> (string=w420:string)
            n161 = Concatenate Strings(w423, " - " ("string"), w420) -> (w422:string)
          }
          frame True {
          }
        }
        n162 = property class="VI"(reference=w403, "Front Panel.Title"=w401) -> ()  [unwired: 1 in, 2 out]
      }
      frame "UI: Resize Tab Content" {
        w432 = u32 16 ("y")
        w428 = 8 ("Position:Left")
        n163 = control-ref of="Tab"() -> (w436:refnum<vi>)
        n164 = invoke class="TabCtl (strict)" method="FitControlToPane"(reference=w436) -> (reference out=w425:refnum<vi>)  [unwired: 2 in, 2 out]
        n165 = property class="TabCtl (strict)"(reference=w425) -> ("PaneHeight"=w434:u32, "PaneWidth"=w433:u32, "TabHeight"=w427:u32)  [unwired: 1 in, 2 out]
        n166 = control-ref of="Broadcast Registry"() -> (w431:refnum<vi>)
        n167 = control-ref of="Error History"() -> (w435:refnum<vi>)
        n168 = Subtract(x=w433, y=w432) -> (x-y=w429:u32)
        n169 = Subtract(x=w434, y=w432) -> (x-y=w430:u32)
        n170 = Add(x=w428, y=w427) -> (x+y=w426:u32)
        n171 = property class="Str"(reference=w435, "Left"=w428, "Top"=w426, "Height"=w430, "Width"=w429) -> ()  [unwired: 1 in, 2 out]
        n172 = property class="Tbl (strict)"(reference=w431, "Left"=w428, "Top"=w426, "Height"=w430, "Width"=w429) -> ()  [unwired: 1 in, 2 out]
      }
      frame "---------- Macro ----------" {
        # "Do not put any code in this frame.\n(It is a separator no-op. You can make a copy of this frame to create a new Macro frame)"
        n173 = call <vilib>:"Add State(s) to Queue__JKI_lib_State_Machine.vi"("State(s) in (\"\")"=w447) -> ("States Out"=w446:string)  [unwired: 14 in]
      }
      frame "Macro: Initialize" {
        w450 = "Data: Initialize\nData: Initialize References\nInitialize Core Data\nUI: Initialize\nUI: Front Panel State >> Open\nUI: Resize Tab Content\nUI: Refresh CSM List\nUI: Update Broadcast Registry\nUI: Update Toolbar"  # Data: Initialize Data: Initialize References Initialize Core Data UI: Initialize UI: Front Panel State >> Open UI: Resize Tab Content UI: Refresh CSM List UI: Update Broadcast Registry UI: Update Toolbar
        # "Initialization Macro\n(This is called once, when the VI starts)"
        n174 = call <vilib>:"Add State(s) to Queue__JKI_lib_State_Machine.vi"("State(s) in Front (\"\")"=w450, "State(s) in (\"\")"=w454) -> ("States Out"=w453:string)  [unwired: 13 in]
      }
      frame "Macro: Exit" {
        # "Exit Macro\n(This is called once, when the VI exits)"
        n175 = Unbundle By Name(w463) -> ("Core.Close Panel on Exit?"=w462:bool)
        n176 = Select(t="UI: Front Panel State >> Close", s=w462, f="") -> (s? t:f=w459:string)
        n177 = call <vilib>:"Add State(s) to Queue__JKI_lib_State_Machine.vi"("State(s) in (\"\")"=w459, "State(s) at Back (\"\")"="Data: Cleanup\nExit") -> ("States Out"=w457:string)  [unwired: 13 in]
        n178 = call <vilib>:"Add State(s) to Queue__JKI_lib_State_Machine.vi"("State(s) in Front (\"\")"=w457, "State(s) in (\"\")"=w466) -> ("States Out"=w465:string)  [unwired: 13 in]
      }
    }
  }
  n179 = call "CSM - Destroy Global Log Event.vi"("Error in"=w4, "CSM Global Log Event"=w10) -> ("Error out"=w3:errorcluster)  [unwired: 9 in]
  n180 = invoke class="VI" method="FP.Close"(error in=w3) -> (error out=w12:errorcluster)  [unwired: 2 in, 2 out]
  n181 = call <vilib>:"Clear Errors.vi"("error in (no error)"=w12) -> ()  [unwired: 5 in, 2 out]
